vi "catalan2.vi"(8 "past":i32[](array[numeric]), 11 "n":i32) -> (2 "ans":i32)   [LabVIEW 2023]
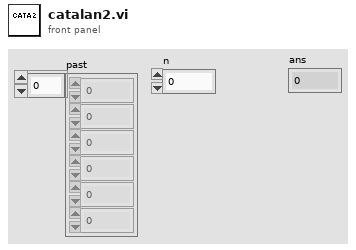
[diagram p1: front panel]
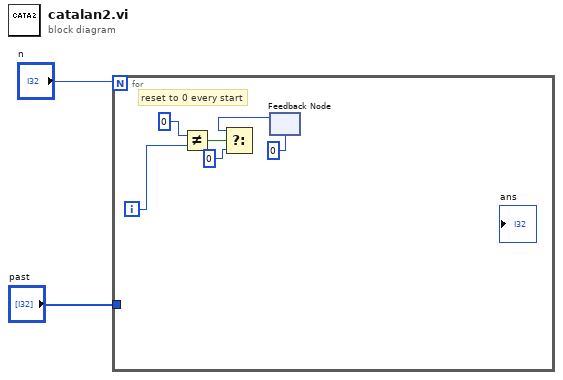
[diagram p0: block diagram]
diagram:
  n1 = for {
    N: "n" -> [_]
    tunnel: "past" -> [_]
    i -> [w4]
    # "reset to 0 every start"
    n2 = Not Equal?(x=0, y=w4) -> (x != y?=w5:bool)
    n3 = feedback-in #1() -> ()  [unwired: 1 out]
    n4 = feedback #1(0) -> (w7:i32)
    n5 = Select(t=w7, s=w5, f=0) -> ()  [unwired: 1 out]
  }
